vi "Temperature.vi"(5 "Set Temperature":sgl, 6 "Action":enum16{"Set Celsius", "Get Temps"}(ring)) -> (0 "Output3":sgl, 1 "Output2":sgl, 2 "Output1":sgl, 3 "Error":bool, 4 "Output4":sgl)   [LabVIEW 2014]
uses:
  globals/AzCamGlobals.vi
panel:
  # "C"
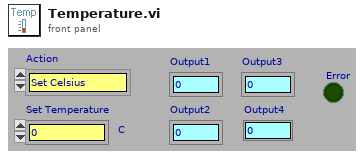
[diagram p1: front panel]
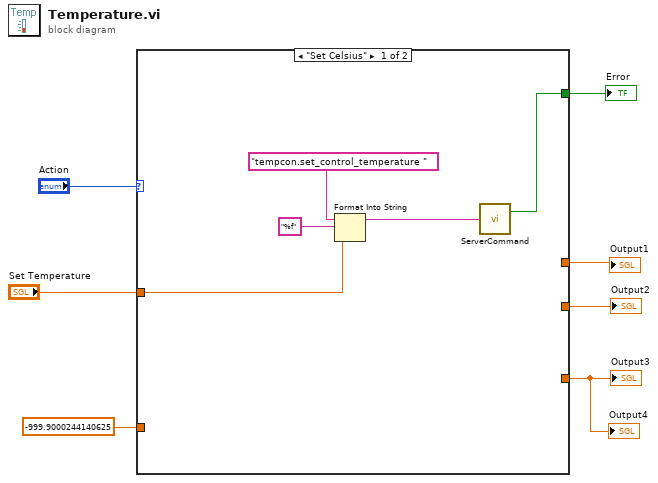
[diagram p0: block diagram]
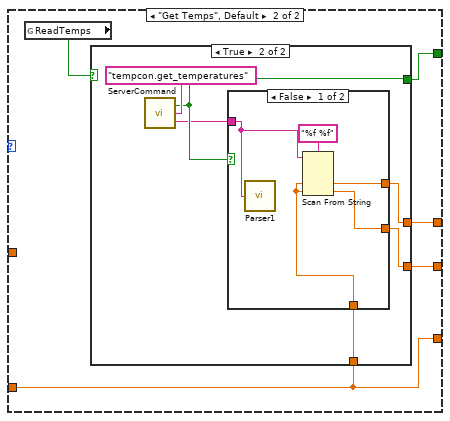
[diagram p2: hidden frame]
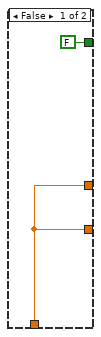
[diagram p3: hidden frame]
diagram:
  n1 = case shown="\"Set Celsius\"" "Action" {
    tunnel: [_ w17] -> w6
    tunnel: "Set Temperature" -> [w12 _]
    tunnel: [_ w16] -> w4
    tunnel: [_ w14] -> w3
    tunnel: [w9 w15] -> w2
    tunnel: sgl -999.9 -> [_ w14]
    frame "Set Celsius" {
      n2 = Format Into String(format string="%f", initial string="tempcon.set_control_temperature " ("Command"), w12) -> (resulting string=w8:string)  [unwired: 1 in, 1 out]
      n3 = call "ServerCommand.vi"("Command"=w8) -> ("Error"=w9:bool)  [unwired: 1 out]
    }
    frame "Get Temps", Default {
      n4 = global read "AzCamGlobals.vi" "ReadTemps"() -> (w13:bool)
      n5 = case shown="True" w13 {
        tunnel: [w19 w25] -> w17
        tunnel: [w19 w23] -> w16
        tunnel: [FALSE ("Error") w22] -> w15
        tunnel: w14 -> [w19 w20]
        frame False {
        }
        frame True {
          n6 = call "ServerCommand.vi"("Command"="tempcon.get_temperatures") -> ("Error"=w22:bool, "Reply"=w21:string)
          n7 = case shown="False" w22 {
            tunnel: [w27 w31] -> w25
            tunnel: [w26 w31] -> w23
            tunnel: w21 -> [w29 _]
            tunnel: w20 -> [w28 w31]
            frame False {
              n8 = call "Parser1.vi"("InputString"=w29) -> ()  [unwired: 6 out]
              n9 = Scan From String(format string="%f %f", input string=w29, default 1=w28, default 2=w28) -> (output 1=w27:sgl, output 2=w26:sgl)  [unwired: 2 in, 3 out]
            }
            frame True {
            }
          }
        }
      }
    }
  }
  "Output1" <- w6
  "Output2" <- w4
  "Error" <- w2
  "Output3" <- w3
  "Output4" <- w3
